vi "readTEDSStatus.vi"(8 "error in (no error)":errorcluster, 11 "ILC in":refnum<class "ILC.lvclass">) -> (0 "error out":errorcluster, 2 "TEDS Status":string, 3 "ILC out":refnum<class "ILC.lvclass">)   [LabVIEW 2015, in "ILCCommon.lvlib" / "ILC.lvclass"]
uses:
  <userlib>/Common/ILC/ILC/ILC.lvclass
  <userlib>/Common/ILC/ILCModelTypedefs/FinalDelimiter.ctl
  <userlib>/Common/ILC/ILC/ILC.lvclass/ILC.ctl
  <userlib>/Common/SerialProtocols/SerialCommunicator/SerialCommunicator.lvclass
  <userlib>/Common/ILC/ILCModelTypedefs/ILCModelTypedefs.lvlib
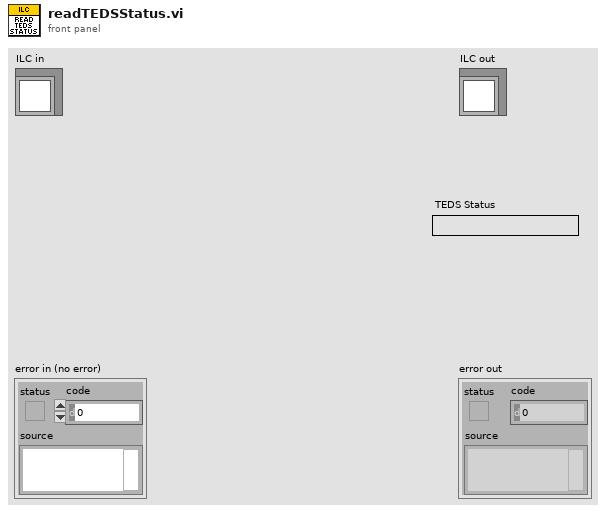
[diagram p1: front panel]
types:
  T1 = typedef "ILCCommon.lvlib/ILCModelTypedefs.lvlib/FinalDelimiter.ctl" = enum16{",", "<CR><LF>"}
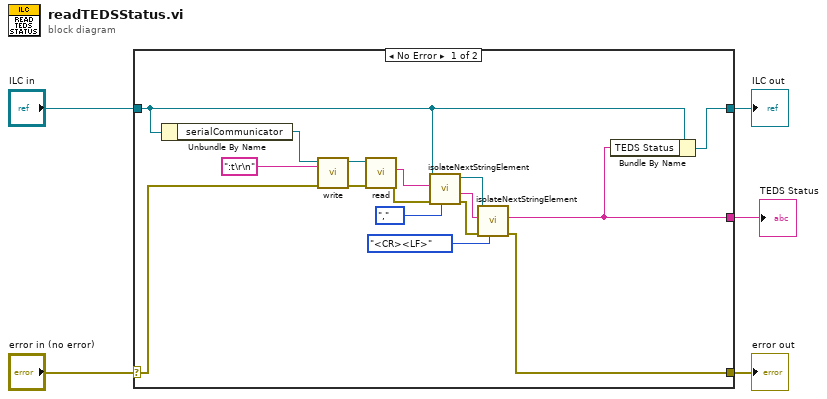
[diagram p0: block diagram]
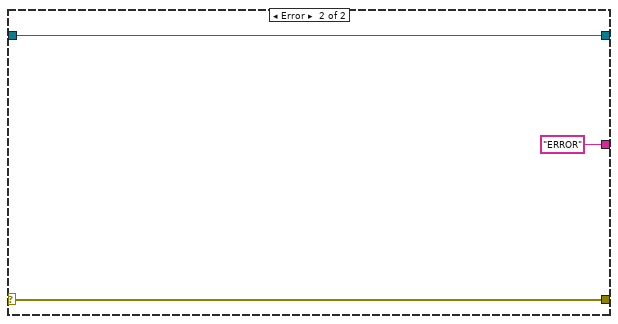
[diagram p2: hidden frame]
diagram:
  n1 = case shown="No Error" "error in (no error)" {
    selector: "error in (no error)" -> [w6 w24]
    tunnel: [w10 w24] -> w4
    tunnel: [w8 w23] -> w2
    tunnel: "ILC in" -> [w9 w23]
    tunnel: [w7 "ERROR" ("extractedSegment")] -> w1
    frame No Error {
      n2 = Unbundle By Name(w9) -> ("serialCommunicator"=w21:refnum<class "SerialCommunicator.lvclass">)
      n3 = call-dynamic "write.vi"("error in (no error)"=w6, "writeString"=":t\r\n", "SerialCommunicator in"=w21) -> ("error out"=w18:errorcluster, "SerialCommunicator out"=w19:refnum<class "SerialCommunicator.lvclass">)  [unwired: 7 in]
      n4 = call-dynamic "read.vi"("error in (no error)"=w18, "SerialCommunicator in"=w19) -> ("error out"=w16:errorcluster, "stringRead"=w17:string)  [unwired: 7 in, 1 out]
      n5 = call <userlib>:"isolateNextStringElement.vi"("Final Delimiter"=FinalDelimiter.",", "error in (no error)"=w16, "inputString"=w17, "ILC in"=w9) -> ("error out"=w12:errorcluster, "remainingString"=w13:string, "ILC out"=w14:refnum<class "ILC.lvclass">)  [unwired: 4 in, 1 out]
      n6 = call <userlib>:"isolateNextStringElement.vi"("Final Delimiter"=FinalDelimiter."<CR><LF>", "error in (no error)"=w12, "inputString"=w13, "ILC in"=w14) -> ("error out"=w10:errorcluster, "extractedSegment"=w7:string)  [unwired: 4 in, 2 out]
      n7 = Bundle By Name(cluster=w9, "TEDS Status"=w7) -> (w8:refnum<class "ILC.lvclass">)
    }
    frame Error {
    }
  }
  "error out" <- w4
  "ILC out" <- w2
  "TEDS Status" <- w1
